vi "Set Velocity Setpoint.vi"(8 "error in (no error)":errorcluster, 10 "CCW Velocity (0 rad/s)":dbl, 11 "DC Motor Controller Sim in":refnum<class "DC Motor Controller Simulator.lvclass">) -> (0 "error out":errorcluster, 3 "DC Motor Controller Sim out":refnum<class "DC Motor Controller Simulator.lvclass">)   [LabVIEW 2019, in "DC Motor Controller Simulator.lvclass"]
doc: "Sets the counterclockwise velocity setpoint of the motor."
uses:
  DC Motor Controller Simulator.lvclass
  <vilib>/robotics/Simulator/Robot Factory/Motor/ODESimulator_Motor.lvclass
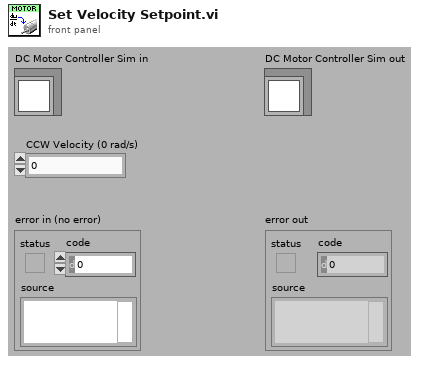
[diagram p1: front panel]
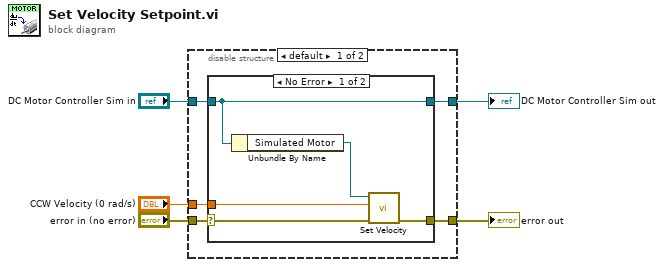
[diagram p0: block diagram]
diagram:
  n1 = disable-structure shown="default" {
    disable-tunnel: "error in (no error)" -> [w10 w18]
    disable-tunnel: "DC Motor Controller Sim in" -> [w9 w19]
    disable-tunnel: [w8 w19] -> w3
    disable-tunnel: [w7 w18] -> w2
    disable-tunnel: "CCW Velocity (0 rad/s)" -> [w6 _]
    frame condition #0 (active) {
      n2 = case shown="No Error" w10 {
        selector: w10 -> [w12 w16]
        tunnel: w9 -> [w15 w17]
        tunnel: [w15 w17] -> w8
        tunnel: [w11 w16] -> w7
        tunnel: w6 -> [w13 _]
        frame No Error {
          n3 = Unbundle By Name(w15) -> ("Simulated Motor"=w14:refnum<class "ODESimulator_Motor.lvclass">)
          n4 = call-dynamic "Set Velocity.vi"("error in (no error)"=w12, "CCW Velocity (0.0 rad/s)"=w13, "Motor in"=w14) -> ("error out"=w11:errorcluster)  [unwired: 7 in, 1 out]
        }
        frame Error {
        }
      }
    }
    frame condition #1 {
    }
  }
  "error out" <- w2
  "DC Motor Controller Sim out" <- w3
